vi "Global Variables.vi"() -> ()   [LabVIEW 2014]
panel:
  in  "B&K update interval":u32=1000
  in  "Omega update interval":u32=1000
  in  "Maximum Current":dbl=1.2
  in  "Maximum Voltage":dbl=73.0
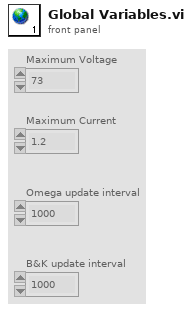
[diagram p1: front panel]
diagram:
